vi "config Keb.vi"(10 "Configurazione keb in":T1) -> (2 "OK Button":bool, 3 "Configurazione keb OUT":T1)   [LabVIEW 2019]
uses:
  ConfigurazioneKeb.ctl
panel:
  in  "Configurazione KEB":T1
  in  "Cancel Button":bool
  in  "OK Button":bool
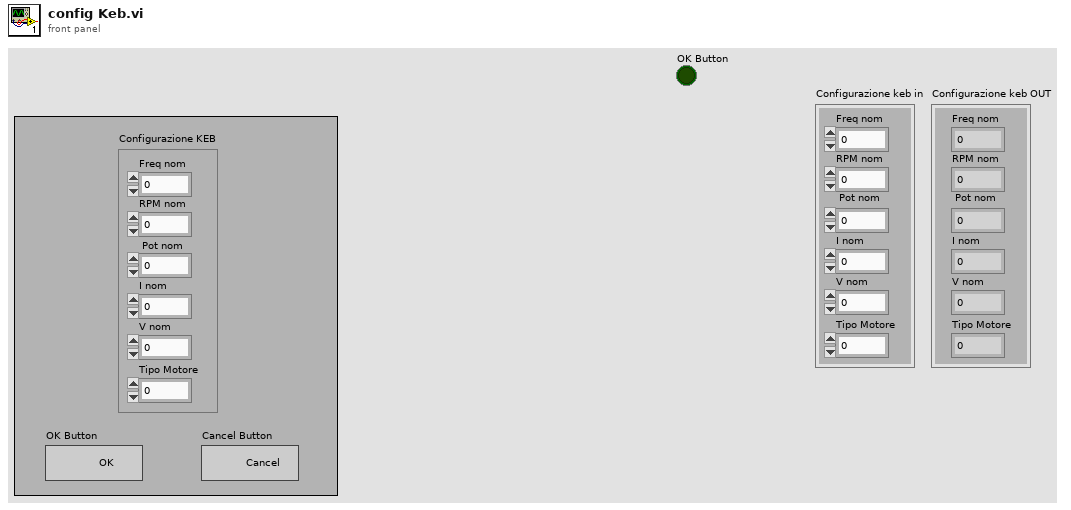
[diagram p1: front panel]
types:
  T1 = typedef "ConfigurazioneKeb.ctl" = cluster{"Freq nom":dbl, "RPM nom":dbl, "Pot nom":dbl, "I nom":dbl, "V nom":dbl, "Rpm max":dbl, "Tipo Motore":dbl}
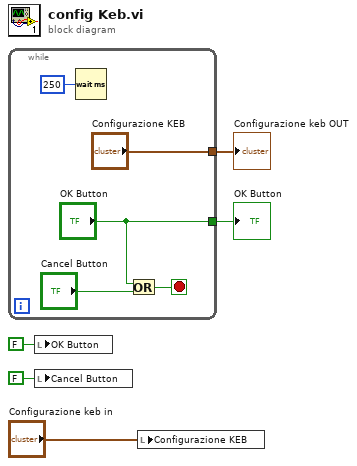
[diagram p0: block diagram]
diagram:
  n1 = while {
    tunnel: ["Configurazione KEB"] -> w1
    tunnel: ["OK Button"] -> w3
    stop <- w8 stop-if-true
    n2 = Wait (ms)(milliseconds to wait=u32 250) -> ()  [unwired: 1 out]
    n3 = Or(x="OK Button", y="Cancel Button") -> (x .or. y?=w8:bool)
  }
  "OK Button" <- w3
  "Configurazione keb OUT" <- w1
  n4 = local write "OK Button"(FALSE ("OK Button")) -> ()
  n5 = local write "Cancel Button"(FALSE ("Cancel Button")) -> ()
  n6 = local write "Configurazione KEB"("Configurazione keb in") -> ()
